vi "Contador.vi"() -> ()   [LabVIEW 2022 SP3]
panel:
  in  "Min":u8
  in  "Max":u8
  in  "Enum":enum16{"Up", "Down"}(ring)
  in  "RESET":bool
  out "Cuenta":u8
  in  "Up/Down":bool
  in  "Start/Stop":bool
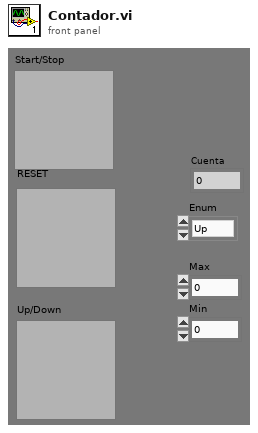
[diagram p1: front panel]
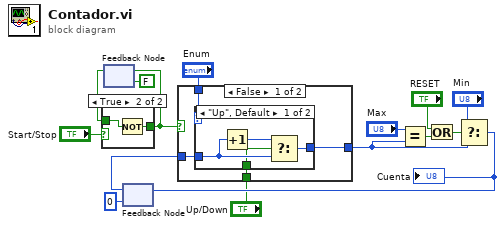
[diagram p0: block diagram]
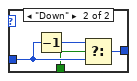
[diagram p3: hidden frame]
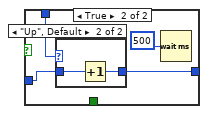
[diagram p4: hidden frame]
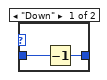
[diagram p5: hidden frame]
diagram:
  n1 = feedback #1(FALSE) -> (w13:bool)
  n2 = case shown="True" "Start/Stop" {
    tunnel: [w16 w18] -> w12
    tunnel: w13 -> [w16 w17]
    frame False {
    }
    frame True {
      n3 = Not(x=w17) -> (.not. x?=w18:bool)
    }
  }
  n4 = feedback-in #1(w12) -> ()
  n5 = feedback #2(u8 0) -> (w15:u8)
  n6 = case shown="False" w12 {
    tunnel: [w22 w32] -> w7
    tunnel: w15 -> [w21 w33]
    tunnel: "Enum" -> [w20 w31]
    tunnel: "Up/Down" -> [w19 _]
    frame False {
      n7 = case shown="\"Up\", Default" w20 {
        tunnel: [w23 w27] -> w22
        tunnel: w21 -> [w25 w29]
        tunnel: w19 -> [w24 w28]
        frame "Up", Default {
          n8 = Increment(x=w25) -> (x+1=w26:u8)
          n9 = Select(t=w26, s=w24, f=w25) -> (s? t:f=w23:u8)
        }
        frame "Down" {
          n10 = Decrement(x=w29) -> (x-1=w30:u8)
          n11 = Select(t=w30, s=w28, f=w29) -> (s? t:f=w27:u8)
        }
      }
    }
    frame True {
      n12 = case shown="\"Up\", Default" w31 {
        tunnel: w33 -> [w35 w38]
        tunnel: [w36 w37] -> w32
        frame "Down" {
          n13 = Decrement(x=w35) -> (x-1=w36:u8)
        }
        frame "Up", Default {
          n14 = Increment(x=w38) -> (x+1=w37:u8)
        }
      }
      n15 = Wait (ms)(milliseconds to wait=u32 500) -> ()  [unwired: 1 out]
    }
  }
  n16 = Equal?(x="Max", y=w7) -> (x = y?=w11:bool)
  n17 = Or(x="RESET", y=w11) -> (x .or. y?=w10:bool)
  n18 = Select(t="Min", s=w10, f=w7) -> (s? t:f=w9:u8)
  "Cuenta" <- w9
  n19 = feedback-in #2(w9) -> ()
